vi "Greatest Common Divisor of p&q (DBL).vi"(0 "p":dbl[](array[numeric]), 1 "order of p":i32, 2 "q":dbl[](array[numeric]), 3 "order of q":i32, 4 "threshold":dbl) -> (5 "greatest common factor":dbl[](array[numeric]), 6 "rest":dbl[](array[numeric]))   [LabVIEW 2020, in "NI_AALPro.lvlib"]
uses:
  NI_AALPro.lvlib
  Remove Zero Threshold Type.ctl
  RMS (DBL).vi
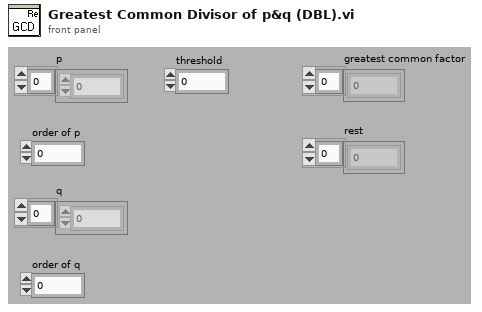
[diagram p1: front panel]
types:
  T1 = typedef "NI_AALPro.lvlib/Remove Zero Threshold Type.ctl" = u16
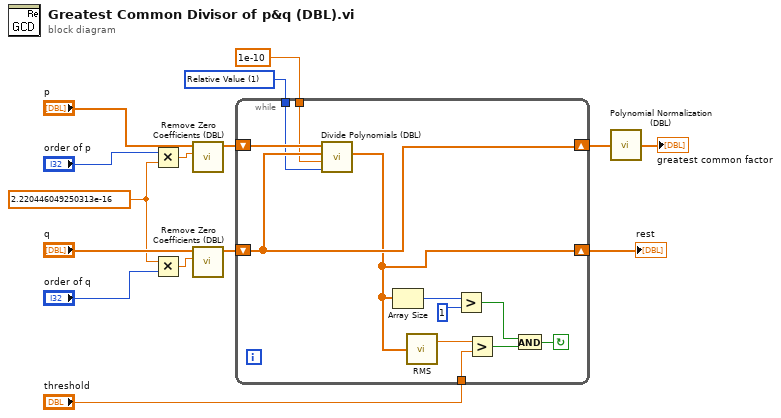
[diagram p0: block diagram]
diagram:
  w2 = T1 1 items=["Absolute Value", "Relative Value"] ("threshold type")
  w8 = 2.220446049250313e-16 ("eps for remove zeros")
  n1 = Multiply(x="order of p", y=w8) -> (x*y=w3:dbl)
  n2 = Multiply(x=w8, y="order of q") -> (x*y=w4:dbl)
  n3 = call "Remove Zero Coefficients (DBL).vi"("threshold"=w3, "P(x) In"="p") -> ("P(x) Out"=w15:dbl[])  [unwired: 7 in, 2 out]
  n4 = call "Remove Zero Coefficients (DBL).vi"("threshold"=w4, "P(x) In"="q") -> ("P(x) Out"=w14:dbl[])  [unwired: 7 in, 2 out]
  n5 = while {
    shift-left: w14 -> [w25]
    shift-right: [w18] -> w13
    shift-left: w15 -> [w27]
    shift-right: [w25] -> w6
    tunnel: "threshold" -> [w23]
    tunnel: w2 -> [w17]
    tunnel: 1e-10 ("threshold") -> [w16]
    stop <- w22 continue-if-true
    n6 = call "Divide Polynomials (DBL).vi"("threshold type"=w17, "threshold"=w16, "Q(x)"=w25, "P(x)"=w27) -> ("Remainder"=w18:dbl[])  [unwired: 5 in, 2 out]
    n7 = Array Size(array=w18) -> (size(s)=w24:i32)
    n8 = call-poly "RMS.vi"("X"=w18) -> ("rms value"=w20:dbl)  [unwired: 1 out]
    n9 = Greater?(x=w24, y=1) -> (0:w21:bool)
    n10 = Greater?(x=w20, y=w23) -> (0:w19:bool)
    n11 = And(x=w21, y=w19) -> (x .and. y?=w22:bool)
  }
  "rest" <- w13
  n12 = call "Polynomial Normalization (DBL).vi"("polynomial"=w6) -> ("normalized polynomial"=→"greatest common factor":dbl[])
